vi "Controller Test Bench (13) - Advanced PID.vi"() -> ()   [LabVIEW 2022 SP3]
uses:
  WhiteNoise.ctl
  <vilib>/sound2/lvsound2.llb/Sound Data Format.ctl
  <vilib>/Utility/error.llb/DialogType.ctl
  <vilib>/sound2/lvsound2.llb/Sampling Mode.ctl
  <vilib>/Analysis/4window.llb/windowTd.ctl
  <vilib>/Analysis/3filter.llb/Filter Passband Type.ctl
  <vilib>/DAQmx/read.llb/DAQmx Read (Analog 1D Wfm NChan NSamp).vi
  <vilib>/DAQmx/write.llb/DAQmx Write (Analog Wfm 1Chan NSamp).vi
  <vilib>/addons/control/pid/pid.llb/PID Advanced (DBL Array).vi
  <vilib>/addons/control/pid/pid.llb/PID Parameter Manager (DBL Array).vi
  <vilib>/addons/control/pid/pid.llb/PID Derivative Action Buffered (DBL Array).vi
  <vilib>/addons/control/pid/pid.llb/PID Get Advanced Error (DBL Array).vi
  <vilib>/addons/control/pid/pid.llb/PID Integral Action Buffered (DBL Array).vi
  <vilib>/addons/control/pid/pid.llb/PID Resize 1D Array.vi
  <vilib>/addons/control/pid/pid.llb/PID Get Advanced Error (DBL).vi
  <vilib>/sound2/lvsound2.llb/Sound Output Set Volume (Single).vi
  <vilib>/Analysis/3filter.llb/Butterworth Filter (DBL).vi
  <vilib>/sound2/lvsound2.llb/Sound Output Write (DBL Single).vi
  <vilib>/DAQmx/create/channels.llb/DAQmx Create Channel (AI-Acceleration-Accelerometer).vi
  <vilib>/DAQmx/configure/timing.llb/DAQmx Timing (Sample Clock).vi
  <vilib>/DAQmx/configure/task.llb/DAQmx Configure Logging (TDMS).vi
  <vilib>/DAQmx/create/channels.llb/DAQmx Create Channel (AO-Voltage-Basic).vi
  <vilib>/DAQmx/miscellaneous.llb/DAQmx Fill In Error Info.vi
  <vilib>/addons/Time Series Analysis/Series Preprocess.llb/TSA Resampling (Waveform).vi
  <vilib>/addons/control/pid/pid.llb/PID (DBL Array).vi
  <vilib>/measure/matone.llb/Harmonic Distortion Analyzer 1 Chan.vi
  <vilib>/measure/maspectr.llb/FFT Spectrum (Mag-Phase) for N Chan.vi
  <vilib>/measure/NI_MAPro.lvlib
  <resource>/objmgr/daqmx.rc
  <vilib>/Analysis/NI_AALPro.lvlib
  <vilib>/measure/NI_MABase.lvlib
  <vilib>/Analysis/NI_AALBase.lvlib
  <vilib>/addons/control/pid/NI_PID_pid.lvlib
  <vilib>/addons/_Advanced Signal Processing/NI_AdvSigProcTSA.lvlib
panel:
  in  "new sampling rate":dbl=1.0
  out "components level":dbl[](array[numeric]) format="%.2p"
  out "THD":dbl format="%.2p"
  out "detected fundamental frequency":dbl format="%.2p"
  in  "Controller Output Rate":dbl=1024.0 format="%0.2f"
  in  "Sample Rate":dbl=1024.0
  in  "Raw Data":bool
  in  "Control":bool
  in  "Folder to save file to":path=path "C:/Users/LAV-UFSC-2023/Documents/LAV-TCC/Dados-Experimentos/Dados-Bancada-LABVIEW"
  in  "Time Out (s)":dbl=60.0
  out "Elapsed Time":i32 caption="Elapsed Time (s)" format="%.2f"
  in  "Tab Control 2":enum32{"Accel0-Only", "Both Accels"}(tab)
  out "Accel0 and Out":waveform(dbl)[](graph)
  out "Accel0, 1 and Out":waveform(dbl)[](graph)
  out "Waveform Graph":waveform(dbl)(graph)
  in  "Output Noise":bool=TRUE
  in  "?":enum32{"White Noise", "Harmonic"}(tab)=enum."Harmonic"
  in  "Cluster":T2={"Seed"=0.0, "Standard Deviation"=1.0, "Reset"=TRUE, "Iterator"=1.0, "Lower Cut-Off 2"=5.0, "Upper Cut-Off 2"=350.0} {"Upper Cut-Off 2" min=5.0 max=350.0 step=10.0; "Lower Cut-Off 2" min=5.0 max=350.0 step=10.0; "Standard Deviation" min=0.001 max=3.5 step=0.05 format="%0.2p"}
  in  "Cluster 2":T3={"Waveform Type"=0, "Frequency"=10.0, "Amplitude"=0.0625} {"Frequency" min=5.0 max=350.0 step=10.0 format="%0.2p"; "Waveform Type" items=["Sine Wave", "Triangle Wave", "Square Wave", "Sawtooth Wave"]; "Amplitude" min=0.001 max=0.3 step=0.05 format="%0.2p"}
  in  "Fs":dbl=44100.0
  in  "#s":dbl=44100.0
  in  "Tab Control":T4(tab)
  in  "setpoint":dbl[](array[numeric])=[0.0] format="%.2f"
  in  "PID gains":T5(array[cluster])=[{"proportional gain (Kc)"=1.0, "integral time (Ti, min)"=0.01, "derivative time (Td, min)"=0.0}] {"derivative time (Td, min)" format="%.3f"; "integral time (Ti, min)" format="%.3f"; "proportional gain (Kc)" step=0.01 format="%.3f"}
  in  "output range":cluster{"output high":dbl, "output low":dbl}[](array[cluster])=[{"output high"=100.0, "output low"=-100.0}] {"output low" format="%.2f"; "output high" format="%.2f"}
  in  "manual control":dbl[](array[numeric])=[0.0] format="%.2f"
  in  "setpoint range":T6(array[cluster])=[{"setpoint high"=100.0, "setpoint low"=0.0}] {"setpoint high" format="%.2f"; "setpoint low" format="%.2f"}
  in  "PID gains":T5(array[cluster])=[{"proportional gain (Kc)"=1.0, "integral time (Ti, min)"=0.01, "derivative time (Td, min)"=0.0}] {"derivative time (Td, min)" format="%.3f"; "integral time (Ti, min)" format="%.3f"; "proportional gain (Kc)" min=0.0 step=0.01 format="%.3f"}
  in  "output range":cluster{"output high":dbl, "output low":dbl}[](array[cluster])=[{"output high"=100.0, "output low"=-100.0}] {"output low" format="%.2f"; "output high" format="%.2f"}
  in  "Setpoint":dbl[](array[numeric])=[0.0] format="%.2f"
  in  "Setpoint":dbl
  in  "Gain":dbl min=0.0 step=0.01
  in  "Upper Cut-Off":dbl=400.0
  in  "Lower Cut-Off":dbl=100.0
  out "Phase 2":cluster{"f0":dbl, "df":dbl, "phase":dbl[]}[](graph)
  out "Mag 2":cluster{"f0":dbl, "df":dbl, "magnitude":dbl[]}[](graph)
  in  "FFT":bool=TRUE
  in  "FFT":bool
  in  "Raw Data":bool=TRUE
  # "Data Acquisition"
  # "Log"
  # "Read"
  # "Output"
  # "Filter"
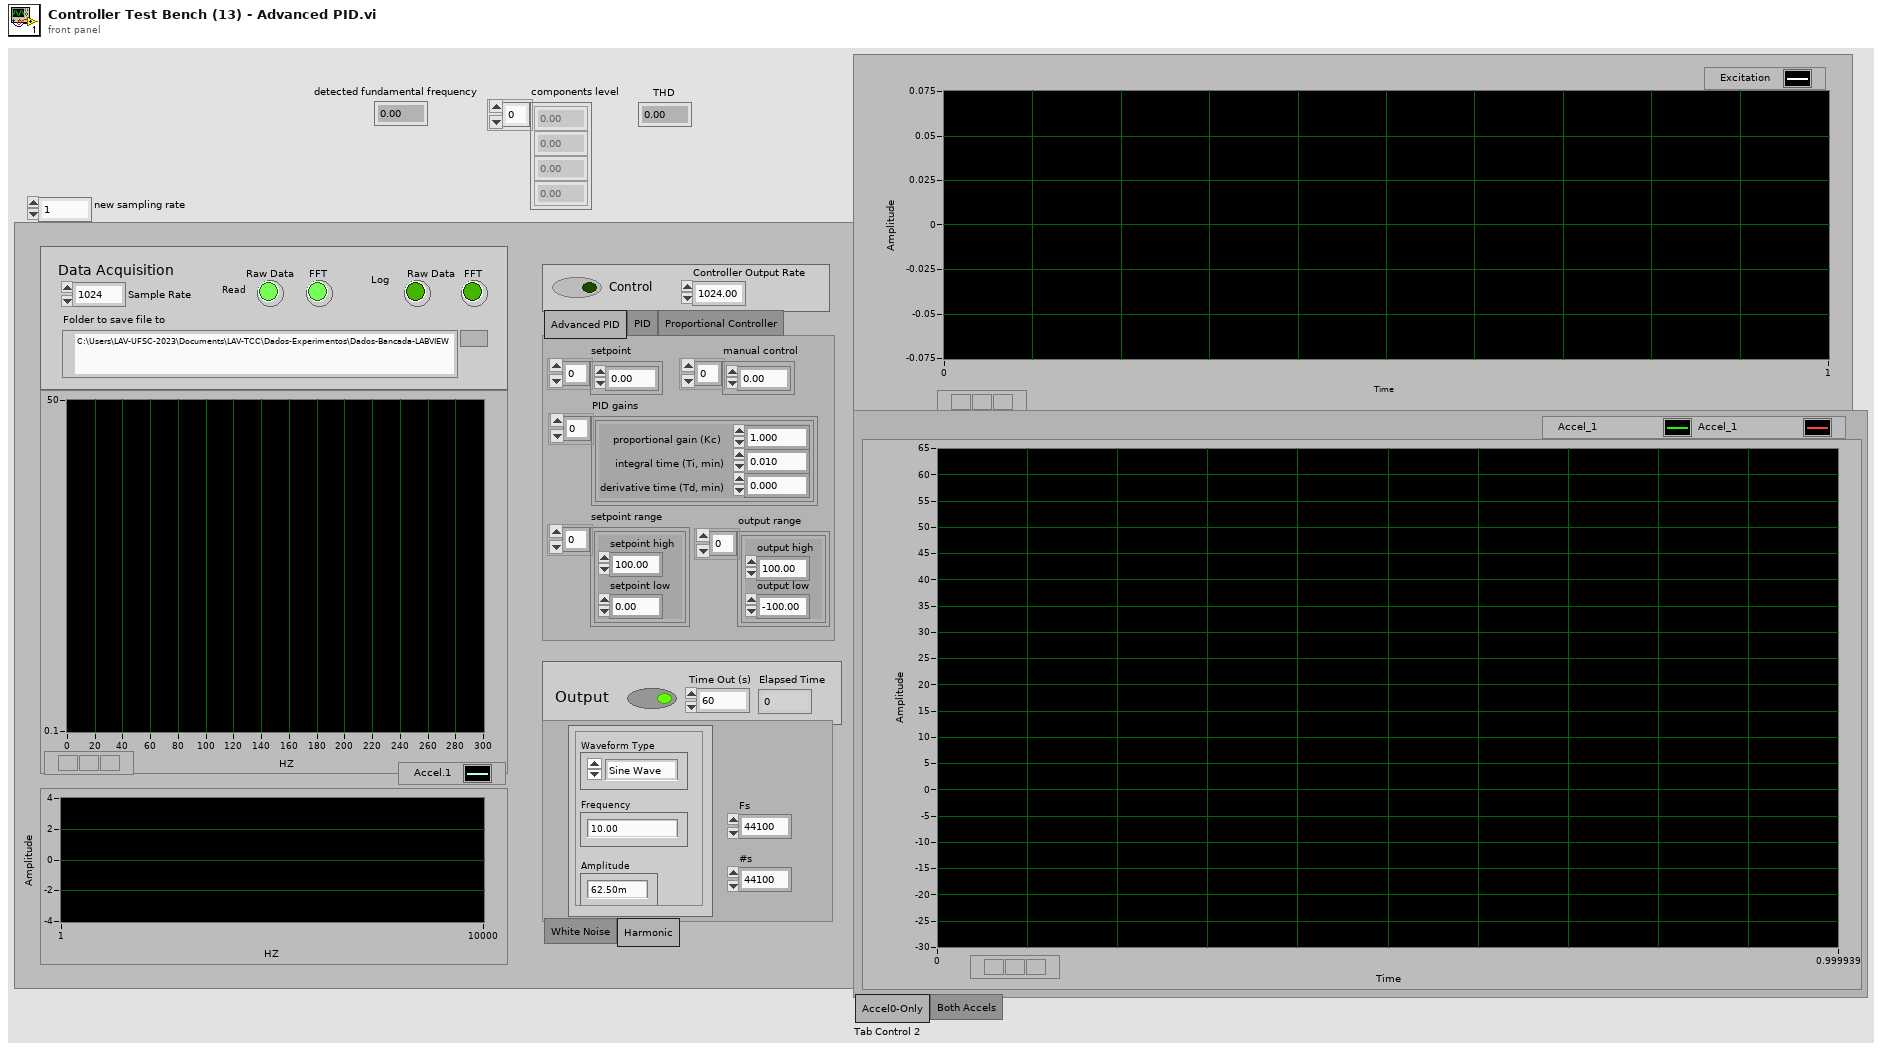
[diagram p1: front panel]
types:
  T1 = typedef "WhiteNoise.ctl" = dbl
  T2 = cluster{"Seed":T1, "Standard Deviation":dbl, "Reset":bool, "Iterator":dbl, "Lower Cut-Off 2":dbl, "Upper Cut-Off 2":dbl}
  T3 = cluster{"Waveform Type":u16, "Frequency":dbl, "Amplitude":dbl}
  T4 = enum32{"Advanced PID", "PID", "Proportional Controller"}
  T5 = cluster{"proportional gain (Kc)":dbl, "integral time (Ti, min)":dbl, "derivative time (Td, min)":dbl}[]
  T6 = cluster{"setpoint high":dbl, "setpoint low":dbl}[]
  T7 = typedef "Sampling Mode.ctl" = i32
  T8 = typedef "DialogType.ctl" = u16
  T9 = typedef "Sound Data Format.ctl" = cluster{"sample rate (S/s)":dbl, "number of channels":i32, "bits per sample":i32}
  T10 = cluster{"dB On (F)":bool, "unwrap phase (F)":bool, "convert to degree (F)":bool}
  T11 = cluster{"averaging mode":enum16{"No averaging", "Vector averaging", "RMS averaging", "Peak hold"}, "weighting mode":enum16{"Linear", "Exponential"}, "number of averages":u32}
  T12 = typedef "NI_AALPro.lvlib/windowTd.ctl" = u32
  T13 = typedef "Sound Output Task ID.ctl" = u32
  T14 = typedef "NI_AALBase.lvlib/Filter Passband Type.ctl" = enum32{"Lowpass", "Highpass", "Bandpass", "Bandstop"}
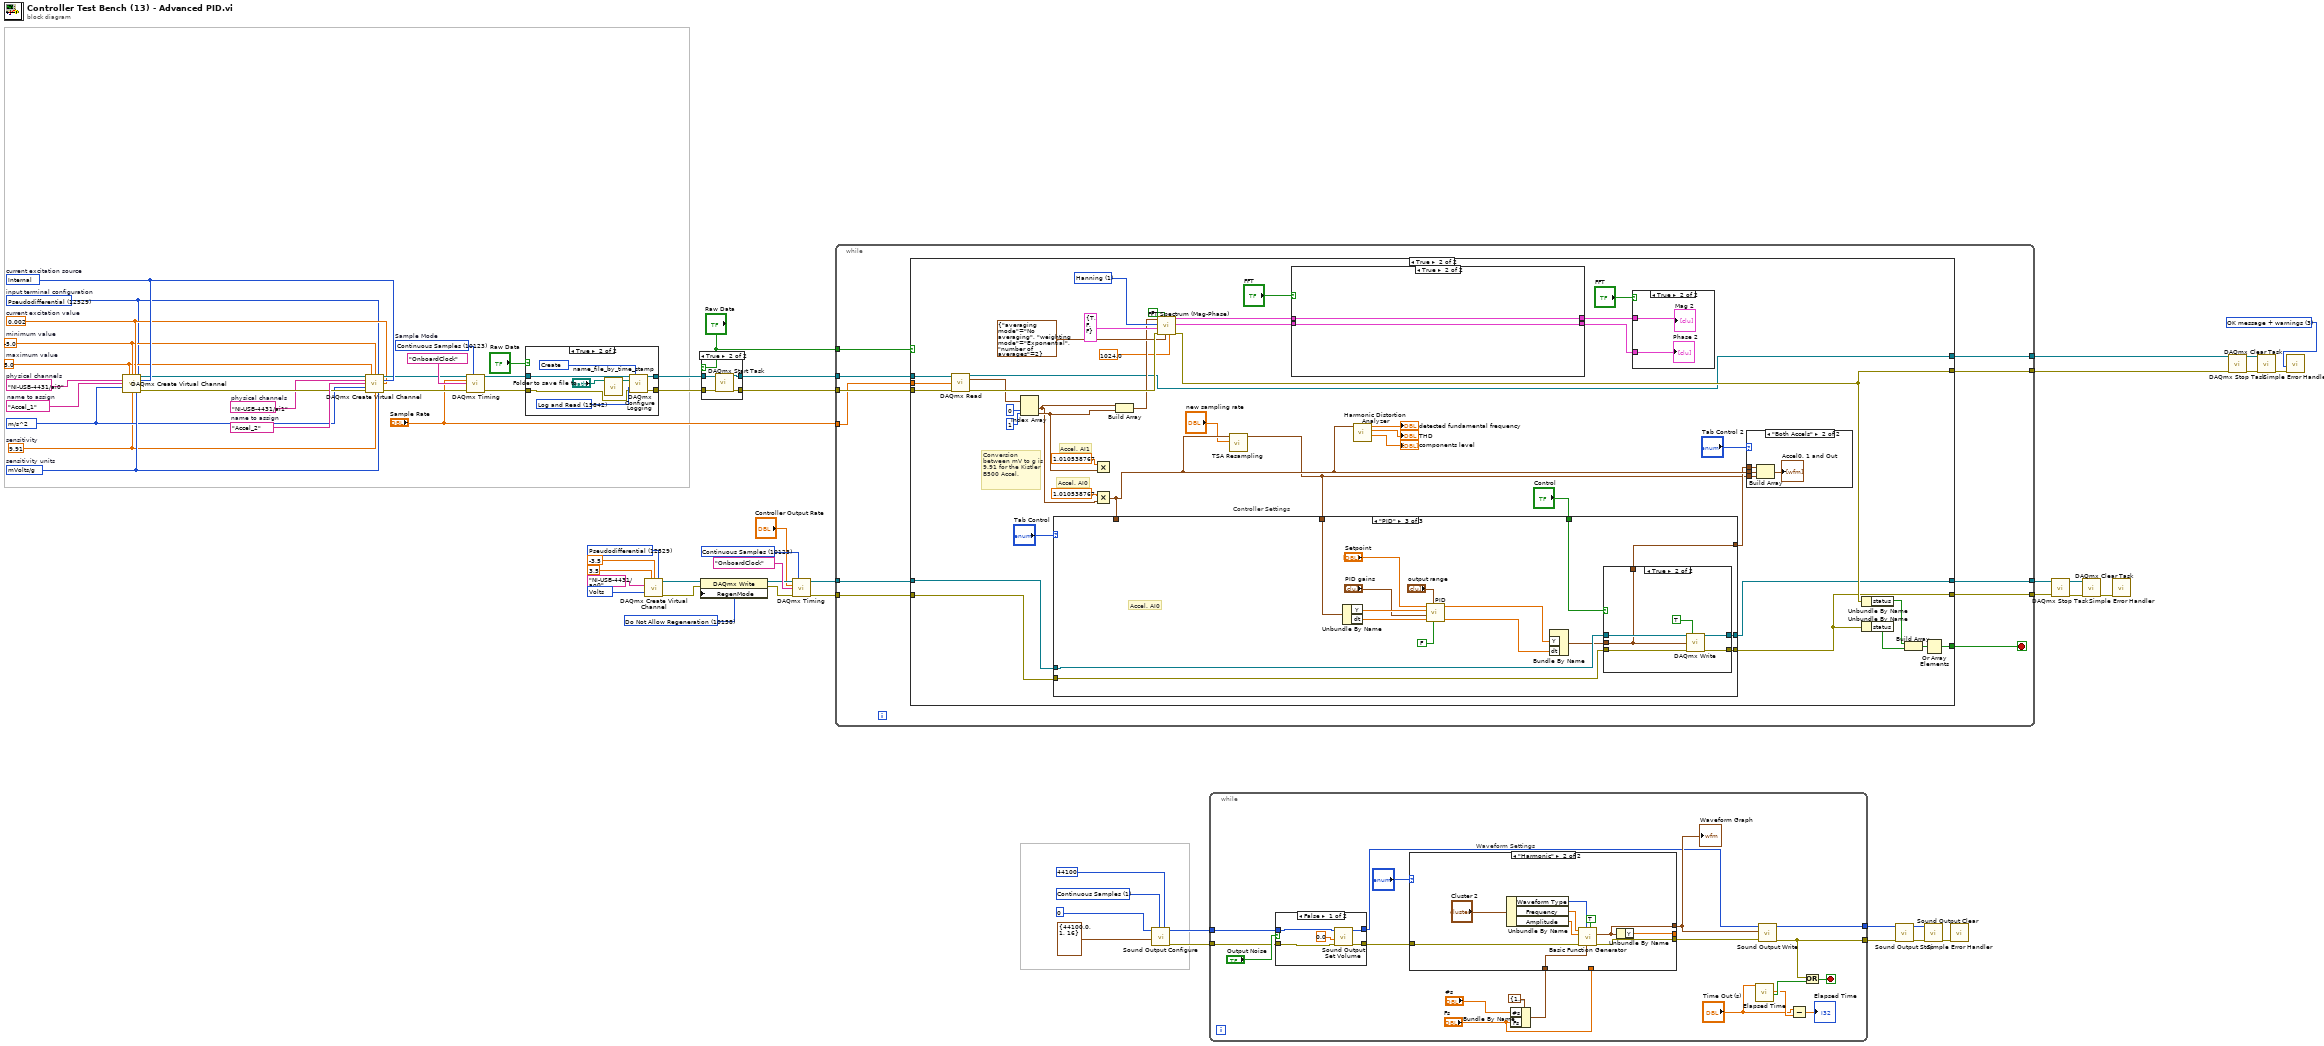
[diagram p0: block diagram]
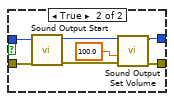
[diagram p2: hidden frame]
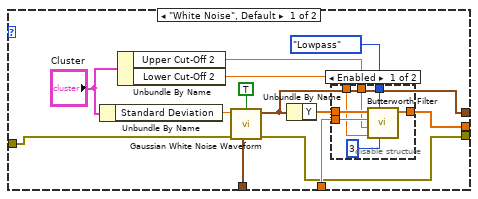
[diagram p3: hidden frame]
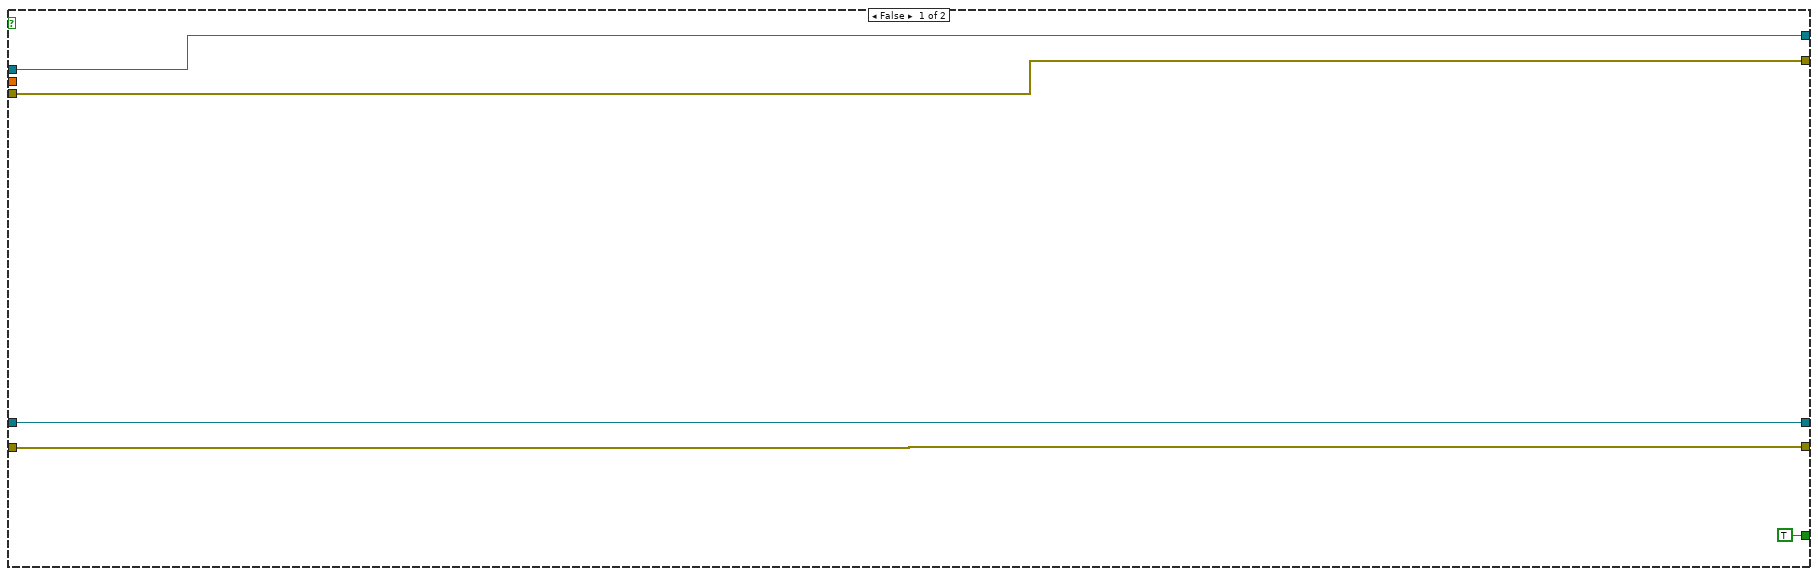
[diagram p5: hidden frame]
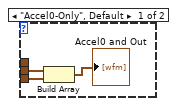
[diagram p6: hidden frame]
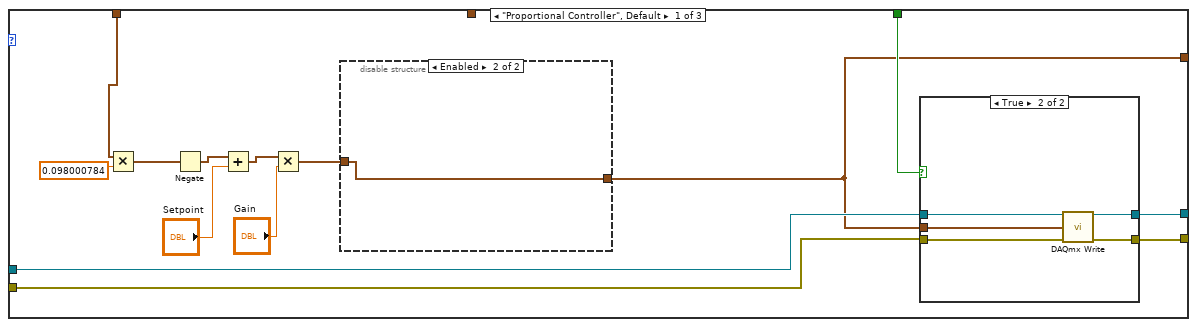
[diagram p7: hidden frame]
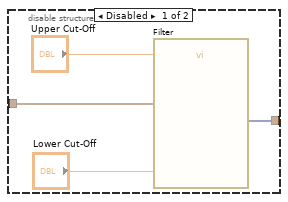
[diagram p8: hidden frame]
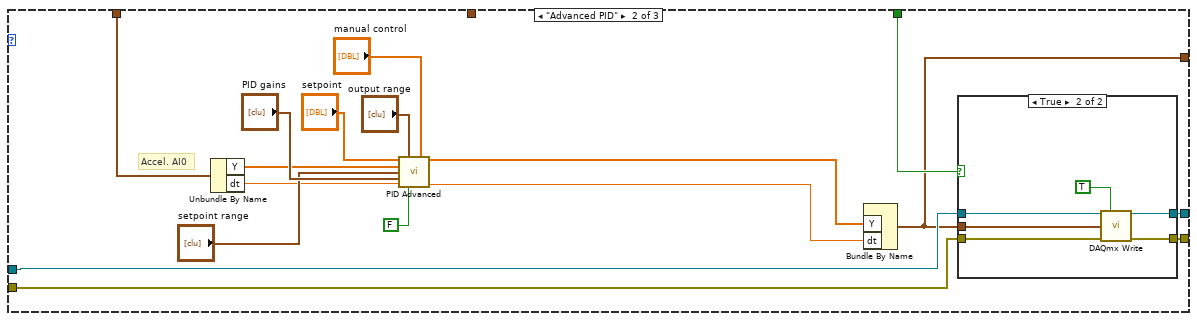
[diagram p10: hidden frame]
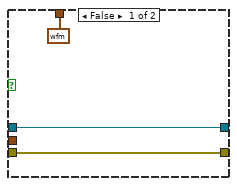
[diagram p12: hidden frame]
diagram:
  w14 = 10123 items=["Finite Samples"=10178, "Continuous Samples"=10123, "Hardware Timed Single Point"=12522] ("sample mode")
  w18 = 10158 items=["Allow Regeneration"=10097, "Do Not Allow Regeneration"=10158] ("RegenMode")
  w23 = 12529 items=["Default"=-1, "RSE"=10083, "Differential"=10106, "Pseudodifferential"=12529] ("output terminal configuration")
  w21 = 10348 items=["Volts"=10348, "From Custom Scale"=10065] ("units")
  w32 = 12470 items=["g"=10186, "m/s^2"=12470, "in/s^2"=12471, "From Custom Scale"=10065] ("units")
  w33 = 12509 items=["mVolts/g"=12509, "Volts/g"=12510]  # sensitivity units
  w31 = 9.91  # sensitivity
  w47 = 0.002  # current excitation value
  w50 = 10200 items=["Internal"=10200, "External"=10167, "None"=10230]  # current excitation source
  w42 = tag "NI-USB-4431/ai0"  # physical channels
  w54 = 10123 items=["Finite Samples"=10178, "Continuous Samples"=10123, "Hardware Timed Single Point"=12522]  # Sample Mode
  w44 = 12529 items=["default"=-1, "RSE"=10083, "NRSE"=10078, "Differential"=10106, "Pseudodifferential"=12529]  # input terminal configuration
  w46 = -5.0  # minimum value
  w45 = 5.0  # maximum value
  w55 = "Accel_1"  # name to assign
  w43 = tag "NI-USB-4431/ai1"  # physical channels
  w52 = "Accel_2"  # name to assign
  w56 = T7 1 items=["Finite Samples", "Continuous Samples"] ("sample mode")
  w57 = T8 3 items=["no dialog", "OK message", "continue or stop message", "OK message + warnings", "continue/stop + warnings"] ("type of dialog (OK msg:1)")
  n1 = call-poly <vilib>:"DAQmx Create Virtual Channel.vi"("maximum value"=w45, "minimum value"=w46, "input terminal configuration"=w44, "physical channels"=w42, "current excitation source"=w50, "name to assign"=w55, "current excitation value"=w47, "units"=w32, "sensitivity"=w31, "sensitivity units"=w33) -> ("task out"=w34:refnum<k21>, "error out"=w51:errorcluster)  [unwired: 4 in]
  n2 = call-poly <vilib>:"DAQmx Create Virtual Channel.vi"("task in"=w34, "maximum value"=w45, "minimum value"=w46, "input terminal configuration"=w44, "physical channels"=w43, "current excitation source"=w50, "name to assign"=w52, "current excitation value"=w47, "units"=w32, "error in"=w51, "sensitivity"=w31, "sensitivity units"=w33) -> ("task out"=w49:refnum<k21>, "error out"=w48:errorcluster)  [unwired: 2 in]
  n3 = call-poly <vilib>:"DAQmx Timing.vi"("task/channels in"=w49, "sample mode"=w54, "rate"="Sample Rate", "source"=tag "OnboardClock" ("Sample Clock Source"), "error in"=w48) -> ("task out"=w30:refnum<k21>, "error out"=w27:errorcluster)  [unwired: 9 in]
  n4 = case shown="True" "Raw Data" {
    tunnel: w30 -> [w66 w71]
    tunnel: [w66 w72] -> w29
    tunnel: [w65 w68] -> w28
    tunnel: w27 -> [w65 w67]
    frame False {
    }
    frame True {
      w73 = 15848 items=["Open"=10437, "Open or Create"=15846, "Create or Replace"=15847, "Create"=15848] ("operation")
      w74 = 15842 items=["Off"=10231, "Log"=15844, "Log and Read"=15842] ("logging mode")
      n5 = call "name_file_by_time_stamp.vi"("Folder to save file to"="Folder to save file to") -> ("New file path"=w70:path)  [unwired: 10 in]
      n6 = call-poly <vilib>:"DAQmx Configure Logging.vi"("task/channels in"=w71, "operation"=w73, "file path"=w70, "logging mode"=w74, "error in"=w67) -> ("task out"=w72:refnum<k21>, "error out"=w68:errorcluster)  [unwired: 9 in]
    }
  }
  n7 = call-poly <vilib>:"DAQmx Create Virtual Channel.vi"("maximum value"=3.5, "minimum value"=-3.5, "output terminal configuration"=w23, "physical channels"=tag "NI-USB-4431/ao0", "units"=w21) -> ("task out"=w17:refnum<k21>, "error out"=w19:errorcluster)  [unwired: 9 in]
  n8 = property class="DAQmx Write"(reference=w17, error in=w19, "RegenMode"=w18) -> (reference out=w15:refnum<k21>, error out=w16:errorcluster)
  n9 = case shown="True" "Raw Data" {
    tunnel: w28 -> [w75 w80]
    tunnel: w29 -> [w76 w79]
    tunnel: [w76 w78] -> w37
    tunnel: [w75 w77] -> w38
    frame False {
    }
    frame True {
      n10 = call <vilib>:"DAQmx Start Task.vi"("task/channels in"=w79, "error in"=w80) -> ("task out"=w78:refnum<k21>, "error out"=w77:errorcluster)  [unwired: 12 in]
    }
  }
  n11 = call-poly <vilib>:"DAQmx Timing.vi"("task/channels in"=w15, "sample mode"=w14, "rate"="Controller Output Rate", "source"=tag "OnboardClock" ("Sample Clock Source"), "error in"=w16) -> ("task out"=w6:refnum<k21>, "error out"=w7:errorcluster)  [unwired: 9 in]
  n12 = while {
    tunnel: "Raw Data" -> [w91]
    tunnel: w7 -> [w90]
    tunnel: w38 -> [w89]
    tunnel: w37 -> [w88]
    tunnel: [w87] -> w36
    tunnel: [w86] -> w35
    tunnel: [w85] -> w8
    tunnel: "Sample Rate" -> [w83]
    tunnel: w6 -> [w82]
    tunnel: [w81] -> w5
    stop <- w84 stop-if-true
    n13 = case shown="True" w91 {
      tunnel: w88 -> [w96 w139]
      tunnel: w89 -> [w95 w138]
      tunnel: [w96 w114] -> w86
      tunnel: [w95 w127] -> w87
      tunnel: w90 -> [w94 w123]
      tunnel: [w94 w122] -> w85
      tunnel: [TRUE w121] -> w84
      tunnel: w83 -> [_ w108]
      tunnel: w82 -> [w92 w106]
      tunnel: [w92 w105] -> w81
      frame False {
      }
      frame True {
        w126 = T12 1 items=["Rectangle"=0, "Hanning"=1, "Hamming"=2, "Blackman-Harris"=3, "Exact Blackman"=4, "Blackman"=5, "Flat Top"=6, "4 Term B-Harris "=7, "7 Term B-Harris"=8, "Low Sidelobe"=9, "Blackman Nuttall"=11, "Triangle"=30, "Bartlett-Hanning"=31, "Bohman"=32, "Parzen"=33, "Welch"=34, "Kaiser"=60, "Dolph-Chebyshev"=61, "Gaussian"=62] ("window")
        # "Accel. AI1"
        # "Accel. AI0"
        # "Conversion between mV to g is 9.91 for the Kistler B500 Accel."
        # "Controller Settings"
        n14 = call-poly <vilib>:"DAQmx Read.vi"("task/channels in"=w139, "number of samples per channel"=w108, "error in"=w138) -> ("task out"=w114:refnum<k21>, "data"=w116:waveform(dbl)[], "error out"=w128:errorcluster)  [unwired: 10 in]
        n15 = Index Array(array=w116, index #1=0 ("index"), index #2=1 ("index")) -> (element #1=w110:waveform(dbl), element #2=w111:waveform(dbl))
        n16 = Multiply(x=1.010538767, y=w111) -> ()  [unwired: 1 out]
        n17 = Multiply(x=1.010538767, y=w110) -> (x*y=w100:waveform(dbl))
        n18 = Build Array(w110, w111) -> (w115:waveform(dbl)[])
        n19 = call-poly <vilib>:"FFT Spectrum (Mag-Phase).vi"("window parameter"=1024.0, "averaging parameters"=T11 {"averaging mode"=enum."No averaging", "weighting mode"=enum."Exponential", "number of averages"=2}, "restart averaging (F)"=FALSE, "error in (no error)"=w128, "view"=T10 {"dB On (F)"=TRUE, "unwrap phase (F)"=FALSE, "convert to degree (F)"=FALSE}, "window"=w126, "time signals"=w115) -> ("error out"=w127:errorcluster, "phases"=w133:cluster{"f0":dbl, "df":dbl, "phase":dbl[]}[], "magnitudes"=w134:cluster{"f0":dbl, "df":dbl, "magnitude":dbl[]}[])  [unwired: 2 out]
        n20 = call-poly <vilib>:"TSA Resampling.vi"("new sampling rate"="new sampling rate", "Xt"=w100) -> ("Xt resampled"=w97:waveform(dbl))  [unwired: 1 in, 8 out]
        n21 = case shown="\"PID\"" "Tab Control" {
          tunnel: w123 -> [w152 w187 w213]
          tunnel: "Control" -> [w148 w186 w212]
          tunnel: [w149 w185 w211] -> w122
          tunnel: w100 -> [w153 w181 _]
          tunnel: w106 -> [w151 w176 w208]
          tunnel: [w150 w175 w207] -> w105
          tunnel: [w147 w173 w199] -> w98
          tunnel: w97 -> [_ _ w198]
          frame "Proportional Controller", Default {
            n22 = Multiply(x=w153, y=0.098000784) -> (x*y=w155:waveform(dbl))
            n23 = Negate(x=w155) -> (-x=w159:waveform(dbl))
            n24 = Add(x=w159, y="Setpoint") -> (x+y=w158:waveform(dbl))
            n25 = Multiply(x=w158, y="Gain") -> (x*y=w156:waveform(dbl))
            n26 = disable-structure shown="Enabled" {
              disable-tunnel: w156 -> [w164 w165]
              disable-tunnel: [w161 w165] -> w147
              frame Disabled {
                n27 = call "Filter"("Lower Cut-Off"="Lower Cut-Off", "Upper Cut-Off"="Upper Cut-Off", "Signal"=w164) -> ("Filtered Signal"=w161:dynamicdata)  [unwired: 7 in, 1 out]
              }
              frame Enabled {
              }
            }
            n28 = case shown="True" w148 {
              tunnel: w152 -> [w167 w172]
              tunnel: [w167 w171] -> w149
              tunnel: w147 -> [_ w168]
              tunnel: w151 -> [w166 w170]
              tunnel: [w166 w169] -> w150
              frame False {
              }
              frame True {
                n29 = call-poly <vilib>:"DAQmx Write.vi"("task/channels in"=w170, "data"=w168, "error in"=w172) -> ("task out"=w169:refnum<k21>, "error out"=w171:errorcluster)  [unwired: 10 in, 1 out]
              }
            }
          }
          frame "Advanced PID" {
            # "Accel. AI0"
            n30 = Unbundle By Name(w181) -> ("Y"=w182:dbl[], "dt"=w178:dbl)
            n31 = call-poly <vilib>:"PID Advanced.vi"("setpoint"="setpoint", "output range"="output range", "manual control"="manual control", "process variable"=w182, "setpoint range"="setpoint range", "PID gains"="PID gains", "dt (s)"=w178, "reinitialize? (F)"=FALSE) -> ("output"=w174:dbl[], "dt out (s)"=w177:dbl)  [unwired: 6 in]
            n32 = Bundle By Name("Y"=w174, "dt"=w177) -> (w173:waveform(dbl))  [unwired: 1 in]
            n33 = case shown="True" w186 {
              tunnel: w187 -> [w191 w197]
              tunnel: [w191 w196] -> w185
              tunnel: w173 -> [_ w195]
              tunnel: w176 -> [w190 w194]
              tunnel: [w190 w193] -> w175
              frame False {
              }
              frame True {
                n34 = call-poly <vilib>:"DAQmx Write.vi"("task/channels in"=w194, "auto start"=TRUE, "data"=w195, "error in"=w197) -> ("task out"=w193:refnum<k21>, "error out"=w196:errorcluster)  [unwired: 9 in, 1 out]
              }
            }
          }
          frame "PID" {
            # "Accel. AI0"
            n35 = Unbundle By Name(w198) -> ("Y"=w204:dbl[], "dt"=w203:dbl)
            n36 = call-poly <vilib>:"PID.vi"("reinitialize? (F)"=FALSE, "output range"="output range", "dt (s)"=w203, "PID gains"="PID gains", "process variable"=w204, "setpoint"="Setpoint") -> ("dt out (s)"=w209:dbl, "output"=w205:dbl[])  [unwired: 4 in]
            n37 = Bundle By Name("Y"=w205, "dt"=w209) -> (w206:waveform(dbl))  [unwired: 1 in]
            n38 = case shown="True" w212 {
              tunnel: w213 -> [w216 w222]
              tunnel: [w216 w221] -> w211
              tunnel: w206 -> [_ w217]
              tunnel: w208 -> [w215 w220]
              tunnel: [w215 w219] -> w207
              tunnel: [waveform(dbl) {"t0"=timestamp(0 s since 1904-01-01), "dt"=1.0, "Y"=[]} w217] -> w199
              frame False {
              }
              frame True {
                n39 = call-poly <vilib>:"DAQmx Write.vi"("task/channels in"=w220, "auto start"=TRUE, "data"=w217, "error in"=w222) -> ("task out"=w219:refnum<k21>, "error out"=w221:errorcluster)  [unwired: 9 in, 1 out]
              }
            }
          }
        }
        n40 = case shown="True" "FFT" {
          tunnel: w134 -> [w223 w226]
          tunnel: w133 -> [w224 w225]
          tunnel: [w224 w225] -> w132
          tunnel: [w223 w226] -> w131
          frame False {
          }
          frame True {
          }
        }
        n41 = call-poly <vilib>:"Harmonic Distortion Analyzer.vi"("signal in"=w100) -> ("components level"=→"components level":dbl[], "THD"=→"THD":dbl, "detected fundamental frequency"=→"detected fundamental frequency":dbl)  [unwired: 5 in, 3 out]
        n42 = case shown="True" "FFT" {
          tunnel: w131 -> [_ w228]
          tunnel: w132 -> [_ w227]
          frame False {
          }
          frame True {
            "Mag 2" <- w228
            "Phase 2" <- w227
          }
        }
        n43 = case shown="\"Both Accels\"" "Tab Control 2" {
          tunnel: w98 -> [_ w146]
          tunnel: w97 -> [w142 w145]
          tunnel: w100 -> [w141 w144]
          frame "Accel0-Only", Default {
            n44 = Build Array(w141, w142) -> (→"Accel0 and Out":waveform(dbl)[])
          }
          frame "Both Accels" {
            n45 = Build Array(w146, w144, w145) -> (→"Accel0, 1 and Out":waveform(dbl)[])
          }
        }
        n46 = Unbundle By Name(w127) -> ("status"=w125:bool)
        n47 = Unbundle By Name(w122) -> ("status"=w130:bool)
        n48 = Build Array(w125, w130) -> (w137:bool[])
        n49 = Or Array Elements(Boolean array=w137) -> (logical OR=w121:bool)
      }
    }
  }
  n50 = call <vilib>:"Sound Output Configure.vi"("number of samples/ch"=44100 ("Number of Samples/ch"), "sample mode"=w56, "sound format"=T9 {"sample rate (S/s)"=44100.0, "number of channels"=1, "bits per sample"=16} ("Sound Format"), "device ID"=u32 0 ("Device ID")) -> ("error out"=w2:errorcluster, "task ID"=w1:T13)  [unwired: 6 in]
  n51 = while {
    tunnel: [w240] -> w10
    tunnel: [w234] -> w9
    tunnel: w2 -> [w232]
    tunnel: w1 -> [w231]
    stop <- w245 stop-if-true
    # "Waveform Settings"
    n52 = case shown="False" "Output Noise" {
      tunnel: w232 -> [w251 w259]
      tunnel: w231 -> [w249 w258]
      tunnel: [w250 w254] -> w230
      tunnel: [w248 w253] -> w229
      frame False {
        n53 = call-poly <vilib>:"Sound Output Set Volume.vi"("error in (no error)"=w251, "volume"=0.0, "task ID"=w249) -> ("error out"=w250:errorcluster, "task ID out"=w248:T13)  [unwired: 7 in]
      }
      frame True {
        n54 = call <vilib>:"Sound Output Start.vi"("error in (no error)"=w259, "task ID"=w258) -> ("error out"=w257:errorcluster, "task ID out"=w255:T13)  [unwired: 8 in]
        n55 = call-poly <vilib>:"Sound Output Set Volume.vi"("error in (no error)"=w257, "volume"=100.0, "task ID"=w255) -> ("error out"=w254:errorcluster, "task ID out"=w253:T13)  [unwired: 7 in]
      }
    }
    n56 = Bundle By Name(cluster=cluster{"Fs":dbl, "#s":dbl} {"Fs"=1000.0, "#s"=1000.0} ("sampling info"), "#s"="#s", "Fs"="Fs") -> (w238:cluster{"Fs":dbl, "#s":dbl})
    n57 = case shown="\"Harmonic\"" "?" {
      tunnel: w238 -> [w272 w289]
      tunnel: w230 -> [w271 w290]
      tunnel: [w261 w288] -> w246
      tunnel: [w262 w282] -> _
      tunnel: "Fs" -> [w265 _]
      tunnel: [w260 w281] -> w235
      frame "White Noise", Default {
        n58 = Unbundle By Name("Cluster") -> ("Standard Deviation"=w268:dbl)
        n59 = Unbundle By Name("Cluster") -> ("Upper Cut-Off 2"=w263:dbl, "Lower Cut-Off 2"=w264:dbl)
        n60 = call <vilib>:"Gaussian White Noise Waveform.vi"("sampling info"=w272, "reset signal"=TRUE, "error in (no error)"=w271, "standard deviation"=w268) -> ("error out"=w261:errorcluster, "signal out"=w260:waveform(dbl))  [unwired: 6 in]
        n61 = Unbundle By Name(w260) -> ("Y"=w266:dbl[])
        n62 = disable-structure shown="Enabled" {
          disable-tunnel: Filter_Passband_Type."Lowpass" ("filter type") -> [w279 _]
          disable-tunnel: w266 -> [w278 w280]
          disable-tunnel: w265 -> [w277 _]
          disable-tunnel: w264 -> [w276 _]
          disable-tunnel: w263 -> [w275 _]
          disable-tunnel: [w273 w280] -> w262
          frame Enabled {
            n63 = call-poly <vilib>:"Butterworth Filter.vi"("order"=3, "filter type"=w279, "low cutoff freq: fl"=w276, "high cutoff freq: fh"=w275, "sampling freq: fs"=w277, "X"=w278) -> ("Filtered X"=w273:dbl[])  [unwired: 2 in, 1 out]
          }
          frame Disabled {
          }
        }
      }
      frame "Harmonic" {
        n64 = Unbundle By Name("Cluster 2") -> ("Waveform Type"=w286:u16, "Frequency"=w285:dbl, "Amplitude"=w284:dbl)
        n65 = call <vilib>:"Basic Function Generator.vi"("reset signal"=TRUE, "sampling info"=w289, "signal type"=w286, "error in (no error)"=w290, "amplitude"=w284, "frequency"=w285) -> ("error out"=w288:errorcluster, "signal out"=w281:waveform(dbl))  [unwired: 3 in, 1 out]
        n66 = Unbundle By Name(w281) -> ("Y"=w282:dbl[])
      }
    }
    "Waveform Graph" <- w235
    n67 = call "Elapsed Time"("Time Target (s)"="Time Out (s)") -> ("Elapsed Time (s)"=w242:dbl, "Time has Elapsed"=w243:bool)  [unwired: 11 in, 6 out]
    n68 = call-poly <vilib>:"Sound Output Write.vi"("error in (no error)"=w246, "data"=w235, "task ID"=w229) -> ("error out"=w240:errorcluster, "task ID out"=w234:T13)  [unwired: 7 in]
    n69 = Subtract(x="Time Out (s)", y=w242) -> (x-y=→"Elapsed Time":dbl)
    n70 = Or(x=w240, y=w243) -> (x .or. y?=w245:bool)
  }
  n71 = call <vilib>:"Sound Output Stop.vi"("error in (no error)"=w10, "task ID"=w9) -> ("error out"=w41:errorcluster, "task ID out"=w40:T13)  [unwired: 8 in]
  n72 = call <vilib>:"Sound Output Clear.vi"("error in (no error)"=w41, "task ID"=w40) -> ("error out"=w39:errorcluster)  [unwired: 9 in]
  n73 = call <vilib>:"Simple Error Handler.vi"("error in (no error)"=w39) -> ()  [unwired: 4 in, 5 out]
  n74 = call <vilib>:"DAQmx Stop Task.vi"("task/channels in"=w5, "error in"=w8) -> ("task out"=w13:refnum<k21>, "error out"=w12:errorcluster)  [unwired: 12 in]
  n75 = call <vilib>:"DAQmx Clear Task.vi"("task in"=w13, "error in"=w12) -> ("error out"=w11:errorcluster)  [unwired: 13 in]
  n76 = call <vilib>:"Simple Error Handler.vi"("error in (no error)"=w11) -> ()  [unwired: 4 in, 5 out]
  n77 = call <vilib>:"DAQmx Stop Task.vi"("task/channels in"=w35, "error in"=w36) -> ("task out"=w60:refnum<k21>, "error out"=w59:errorcluster)  [unwired: 12 in]
  n78 = call <vilib>:"DAQmx Clear Task.vi"("task in"=w60, "error in"=w59) -> ("error out"=w61:errorcluster)  [unwired: 13 in]
  n79 = call <vilib>:"Simple Error Handler.vi"("type of dialog (OK msg:1)"=w57, "error in (no error)"=w61) -> ()  [unwired: 3 in, 5 out]
